vi "MB Ethernet Master Query.vi"(7 "MBAP Header":T1, 8 "error in (no error)":errorcluster, 10 "Modbus Command":T2={"Function Code"=1, "Starting Address"=0, "Quantity"=0, "Data"=[], "Discrete"=[]} {"Function Code" items=["Read Coils"=1, "Read Discrete Inputs"=2, "Read Holding Registers"=3, "Read Input Registers"=4, "Write Single Coil"=5, "Write Single Register"=6, "Read Exception Status"=7, "Write Multiple Coils"=15, "Write Multiple Registers"=16]}, 11 "TCP in":refnum<class "TCP.lvclass">) -> (0 "error out":errorcluster, 1 "Exception Code":u8 format="%.0x", 2 "Registers":cluster{"Registers":u16[], "Discrete":bool[]}, 3 "TCP out":refnum<class "TCP.lvclass">)   [LabVIEW 2019, in "NI_modbus_upd.lvlib"]
uses:
  NI_modbus_upd.lvlib
  Ctl/MB Modbus Command.ctl
  TCP/TCP.lvclass
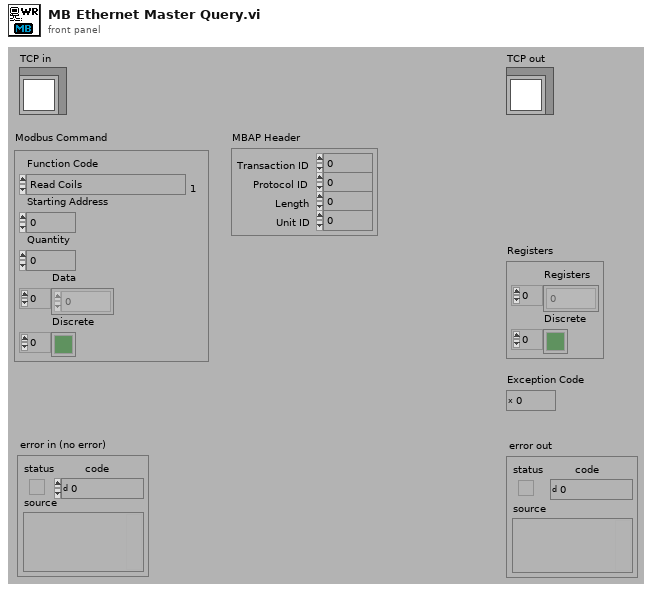
[diagram p1: front panel]
types:
  T1 = cluster{"Transaction ID":u16, "Protocol ID":u16, "Length":u16, "Unit ID":u8}
  T2 = typedef "NI_modbus_upd.lvlib/MB Modbus Command.ctl" = cluster{"Function Code":u8, "Starting Address":u16, "Quantity":u16, "Data":u16[], "Discrete":bool[]}
  T3 = typedef "NI_modbus_upd.lvlib/MB Modbus Data Unit.ctl" = cluster{"function":T4, "Data":u8[]}
  T4 = typedef "NI_modbus_upd.lvlib/Function.ctl" = u8
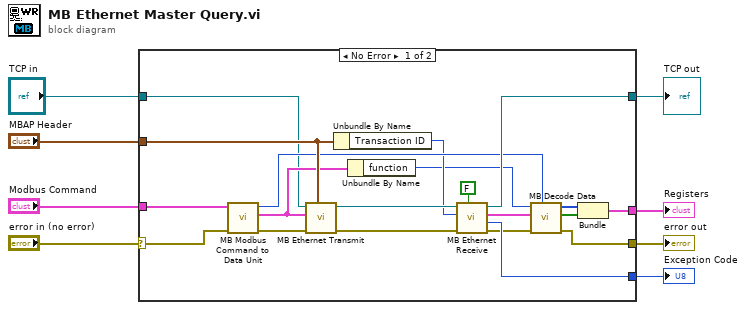
[diagram p0: block diagram]
diagram:
  n1 = case shown="No Error" "error in (no error)" {
    selector: "error in (no error)" -> [w16 w30]
    tunnel: [w27 _] -> w8
    tunnel: [w24 w30] -> w5
    tunnel: [w28 w29] -> w1
    tunnel: "Modbus Command" -> [w15 _]
    tunnel: [w25 _] -> w6
    tunnel: "MBAP Header" -> [w17 _]
    tunnel: "TCP in" -> [w9 w29]
    frame No Error {
      n2 = call "MB Modbus Command to Data Unit.vi"("error in (no error)"=w16, "Modbus Command"=w15) -> ("error out"=w10:errorcluster, "Modbus Data Unit"=w13:T3, "Quantity"=w14:u16)  [unwired: 7 in]
      n3 = call "MB Ethernet Transmit.vi"("MBAP Header"=w17, "error in (no error)"=w10, "Modbus Data Unit"=w13, "TCP in"=w9) -> ("error out"=w20:errorcluster, "TCP out"=w21:refnum<class "TCP.lvclass">)  [unwired: 6 in]
      n4 = Unbundle By Name(w17) -> ("Transaction ID"=w12:u16)
      n5 = Unbundle By Name(w13) -> ("function"=w11:T4)
      n6 = call "MB Ethernet Receive.vi"("Slave"=FALSE, "error in (no error)"=w20, "Transaction ID WR"=w12, "TCP in"=w21) -> ("error out"=w18:errorcluster, "Exception Code"=w27:u8, "Modbus Data Unit"=w26:T3, "TCP out"=w28:refnum<class "TCP.lvclass">)  [unwired: 3 in, 1 out]
      n7 = call "MB Decode Data.vi"("Quantity"=w14, "error in (no error)"=w18, "Response MDU"=w26, "Function Code"=w11) -> ("error out"=w24:errorcluster, "Discrete"=w22:bool[], "Registers"=w23:u16[])  [unwired: 5 in]
      n8 = Bundle("Registers"=w23, "Discrete"=w22) -> (w25:cluster{"Registers":u16[], "Discrete":bool[]})  [unwired: 1 in]
    }
    frame Error {
    }
  }
  "error out" <- w5
  "Exception Code" <- w8
  "Registers" <- w6
  "TCP out" <- w1
